vi "Waiting for rising or falling edge of the signal.vi"(7 "Time to wait":i32=999, 8 "error in":errorcluster, 9 "Rising/Falling edge":bool, 10 "Variable name":string, 11 "UTP IO Session in":T1) -> (0 "error out":errorcluster, 2 "ExpiredTimeToWait?":bool, 3 "UTP IO Session out":T1)   [LabVIEW 2023, in "Actuators.lvlib"]
doc: "True for the Rising Edge\nFalse for the Falling Edge\nIf \"TimeToWait\" has expired, that means we didn't catch rising/falling edge\nPeriod for reading is 10ms"
uses:
  Actuators.lvlib
  <vilib>/Noffz/UTP IO/UTP IO Library/Typedefs/Session Handle.ctl
  <vilib>/Noffz/UTP IO/UTP IO Library/UTP IO Pool Session.lvclass
  <vilib>/Noffz/UTP IO/UTP IO Library/methods/poly/plc/Read PLC Variable (Boolean).vi
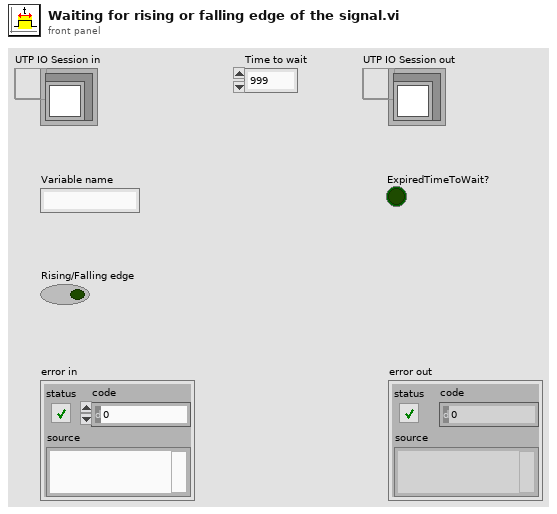
[diagram p1: front panel]
types:
  T1 = typedef "UTP IO Library.lvlib/UTP IO Pool Session.lvclass/Session Handle.ctl" = refnum<data-value>
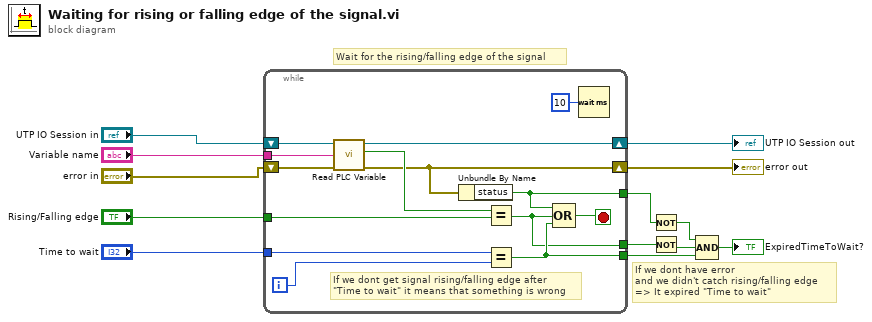
[diagram p0: block diagram]
diagram:
  # "If we dont have error\nand we didn't catch rising/falling edge\n=> It expired \"Time to wait\""
  # "Wait for the rising/falling edge of the signal"
  n1 = while {
    tunnel: "Variable name" -> [w23]
    tunnel: "Rising/Falling edge" -> [w22]
    shift-right: [w25] -> w2
    shift-left: "UTP IO Session in" -> [w27]
    shift-right: [w21] -> w11
    shift-left: "error in" -> [w26]
    tunnel: [w17] -> w9
    tunnel: [w16] -> w8
    tunnel: [w15] -> w5
    tunnel: "Time to wait" -> [w14]
    i -> [w19]
    stop <- w18 stop-if-true
    # "If we dont get signal rising/falling edge after \n\"Time to wait\" it means that something is wrong"
    n2 = call-poly <vilib>:"Read PLC Variable.vi"("error in (no error)"=w26, "variable name"=w23, "UTP IO Session in"=w27) -> ("error out"=w21:errorcluster, "value"=w24:bool, "UTP IO Session out"=w25:T1)  [unwired: 6 in]
    n3 = Unbundle By Name(w21) -> ("status"=w16:bool)
    n4 = Equal?(x=w24, y=w22) -> (x = y?=w15:bool)
    n5 = Equal?(x=w14, y=w19) -> (x = y?=w17:bool)
    n6 = Compound Arithmetic op=OR(w16, w15, w17) -> (w18:bool)
    n7 = Wait (ms)(milliseconds to wait=u32 10) -> ()  [unwired: 1 out]
  }
  "error out" <- w11
  "UTP IO Session out" <- w2
  n8 = Not(x=w8) -> (.not. x?=w7:bool)
  n9 = Not(x=w5) -> (.not. x?=w6:bool)
  n10 = Compound Arithmetic op=AND(w7, w6, w9) -> (→"ExpiredTimeToWait?":bool)
